vi "WPI_IMU_ADIS16448_SPIDelay.vi"(8 "error in":errorcluster, 11 "SPIDevRef in":T1) -> (0 "error out":errorcluster, 3 "SPIDevRef out":T1)   [LabVIEW 2015, in "FRC_ADIS16448_IMU.lvlib"]
uses:
  FRC_ADIS16448_IMU.lvlib
  <vilib>/Rock Robotics/WPI/SPI/WPI_SPIDevRef.ctl
  <vilib>/Rock Robotics/SystemInterfaces/spilib/spi_bus.ctl
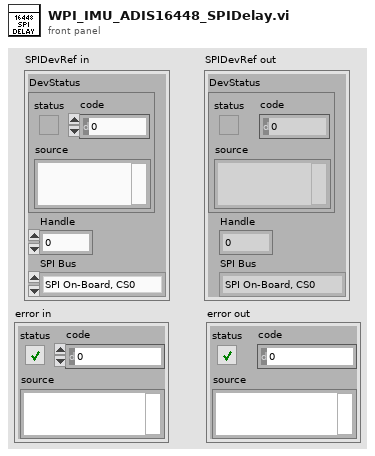
[diagram p1: front panel]
types:
  T1 = typedef "WPI_SPIDevRef.ctl" = cluster{"DevStatus":errorcluster, "Handle":i32, "SPI Bus":T2}
  T2 = typedef "spi_bus.ctl" = enum16{"SPI On-Board, CS0", "SPI On-Board, CS1", "SPI On-Board, CS2", "SPI On-Board, CS3", "SPI MXP", "Invalid"}
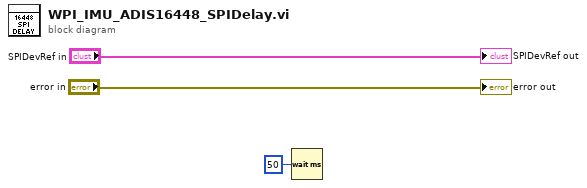
[diagram p0: block diagram]
diagram:
  n1 = Wait (ms)(milliseconds to wait=u32 50) -> ()  [unwired: 1 out]
  "SPIDevRef out" <- "SPIDevRef in"
  "error out" <- "error in"
